vi "Add New UI Reference.vi"(8 "error in (no error)":errorcluster, 9 "Name":string, 10 "VI Refnum":refnum<vi>, 11 "UI Reference Wrapper in":refnum<class "UI Reference Wrapper.lvclass">) -> (0 "error out":errorcluster, 3 "UI Reference Wrapper out":refnum<class "UI Reference Wrapper.lvclass">)   [LabVIEW 2020, in "UI Reference Wrapper.lvclass"]
uses:
  UI Reference Wrapper.lvclass
  UI Reference Wrapper.lvclass/UI Reference Wrapper.ctl
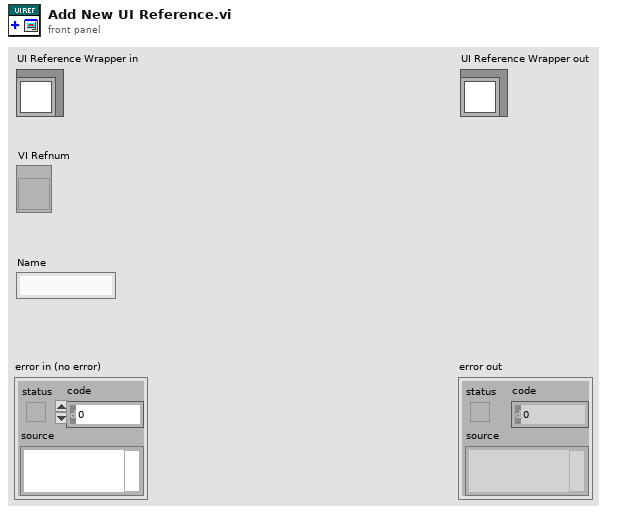
[diagram p1: front panel]
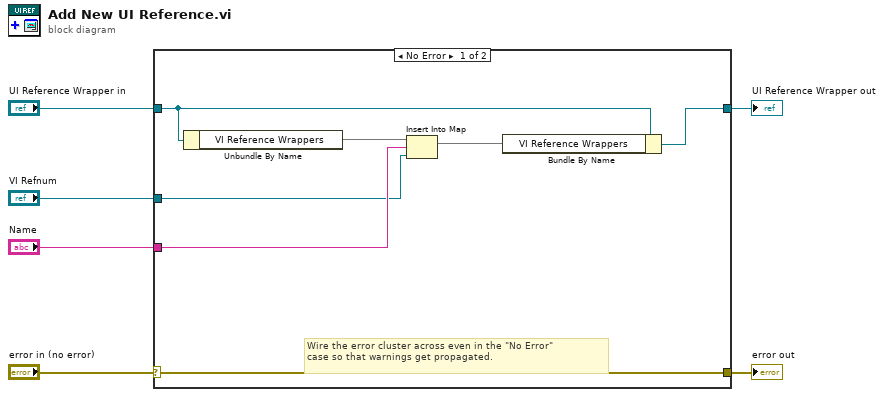
[diagram p0: block diagram]
diagram:
  n1 = case shown="No Error" "error in (no error)" {
    selector: "error in (no error)" -> [w13 w15]
    tunnel: [w13 w15] -> w5
    tunnel: [w11 w14] -> w3
    tunnel: "UI Reference Wrapper in" -> [w12 w14]
    tunnel: "VI Refnum" -> [w7 _]
    tunnel: "Name" -> [w8 _]
    frame No Error {
      # "Wire the error cluster across even in the \"No Error\"\ncase so that warnings get propagated."
      n2 = Unbundle By Name(w12) -> ("VI Reference Wrappers"=w10:map{string, refnum<vi>})
      n3 = Insert Into Map(map in=w10, key=w8, value=w7) -> (map out=w9:map{string, refnum<vi>})  [unwired: 2 out]
      n4 = Bundle By Name(cluster=w12, "VI Reference Wrappers"=w9) -> (w11:refnum<class "UI Reference Wrapper.lvclass">)
    }
    frame Error {
    }
  }
  "error out" <- w5
  "UI Reference Wrapper out" <- w3
